vi "MagDir to MotorOut.vi"(8 "Fwd. Dir?":bool, 10 "Input":i16) -> (2 "Output":i16)   [LabVIEW 2013, in "ProcessorHelperFunctions.lvlib"]
uses:
  ProcessorHelperFunctions.lvlib
panel:
  # "assumes input from 0 to 512, 255=stop"
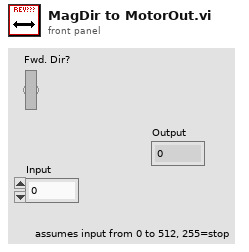
[diagram p1: front panel]
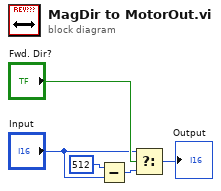
[diagram p0: block diagram]
diagram:
  n1 = Subtract(x=512, y="Input") -> (x-y=w4:i32)
  n2 = Select(t="Input", s="Fwd. Dir?", f=w4) -> (s? t:f=→"Output":i32)
